vi "ma_SML RT Baseband Zoom FFT (real input).vi"(0 "x [V]":dbl[](array[numeric]) format="%.2f", 5 "zoom settings":T2={"zoom"=1, "stop band attenuation"=enum."120 dB", "alias protect in final transition"=FALSE, "oversampling ratio"=1.0} {"oversampling ratio" format="%.2f"; "zoom" min=0}, 7 "FFT settings":T3={"window"=1, "Window Size"=1024, "FFT Size"=1024, "%overlap"=0.0} {"%overlap" min=0.0 max=100.0 format="%.2f"; "window" items=["Rectangle"=0, "Hanning"=1, "Hamming"=2, "Blackman-Harris"=3, "Exact Blackman"=4, "Blackman"=5, "Flat Top"=6, "4 Term B-Harris "=7, "7 Term B-Harris"=8, "Low Sidelobe"=9, "Blackman Nuttall"=11, "Triangle"=30, "Bartlett-Hanning"=31, "Bohman"=32, "Parzen"=33, "Welch"=34, "Kaiser"=60, "Dolph-Chebyshev"=61, "Gaussian"=62]}, 11 "error in (no error)":errorcluster, 12 "reset?":bool) -> (4 "FFT{X} [Vrms]":cdb[](array[numeric]) format="%.2f", 6 "time data":dbl[](array[numeric]) format="%.2f", 8 "spectral info":T1 {"window" items=["Rectangle"=0, "Hanning"=1, "Hamming"=2, "Blackman-Harris"=3, "Exact Blackman"=4, "Blackman"=5, "Flat Top"=6, "4 Term B-Harris "=7, "7 Term B-Harris"=8, "Low Sidelobe"=9, "Blackman Nuttall"=11, "Triangle"=30, "Bartlett-Hanning"=31, "Bohman"=32, "Parzen"=33, "Welch"=34, "Kaiser"=60, "Dolph-Chebyshev"=61, "Gaussian"=62]}, 10 "spectrum ready?":bool, 14 "filter transition length":i32=1 min=0, 15 "error out":errorcluster)   [LabVIEW 2020, in "NI_MAPro.lvlib"]
uses:
  NI_MAPro.lvlib
  ma_sml_Spectral Info.ctl
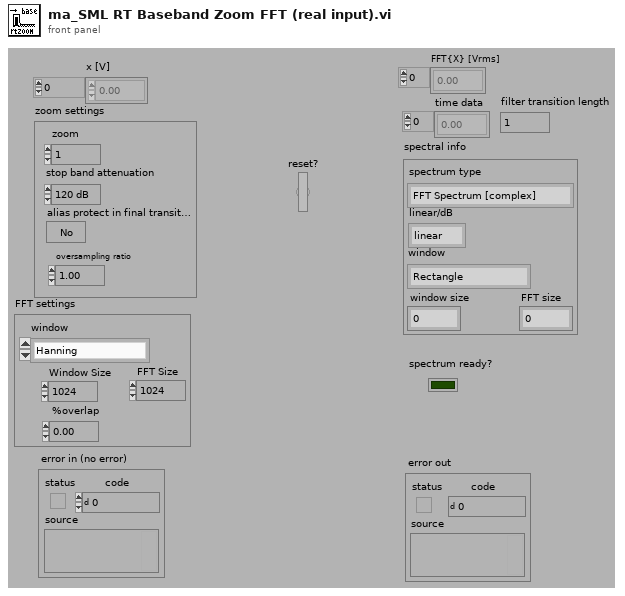
[diagram p1: front panel]
types:
  T1 = typedef "NI_MAPro.lvlib/ma_sml_Spectral Info.ctl" = cluster{"spectrum type":enum16{"FFT Spectrum [complex]", "Amplitude [Magnitude]", "Power [Magnitude^2]", "Cross Spectrum [complex]", "Frequency Response [Complex]"}, "linear/dB":enum16{"linear", "dB"}, "window":u16, "window size":i32, "FFT size":i32}
  T2 = cluster{"zoom":i32, "stop band attenuation":enum16{"84 dB", "96 dB", "120 dB"}, "alias protect in final transition":bool, "oversampling ratio":dbl}
  T3 = cluster{"window":u16, "Window Size":i32, "FFT Size":i32, "%overlap":dbl}
  T4 = cluster{"zoom":bool, "stop band attenuation":bool, "alias protect in final transition":bool, "oversampling ratio":bool}
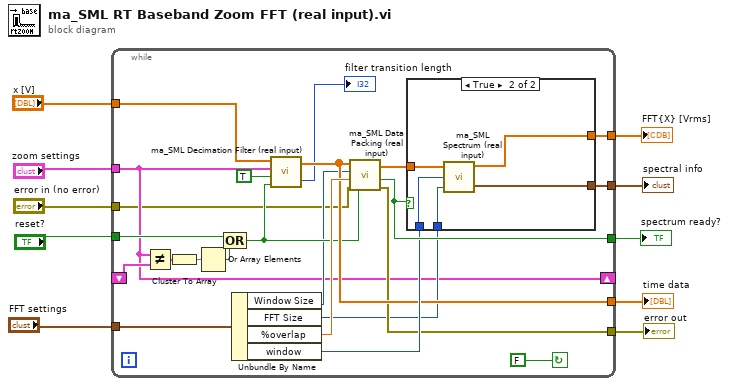
[diagram p0: block diagram]
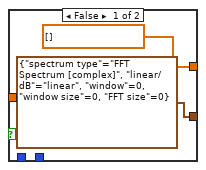
[diagram p2: hidden frame]
diagram:
  n1 = while {
    tunnel: [w11] -> w1
    tunnel: "reset?" -> [w26]
    tunnel: "error in (no error)" -> [w12]
    tunnel: "x [V]" -> [w13]
    tunnel: "FFT settings" -> [w14]
    tunnel: "zoom settings" -> [w15]
    tunnel: [w22] -> w7
    tunnel: [w23] -> w8
    tunnel: [w24] -> w9
    shift-left: _ -> [w25]
    shift-right: [w15] -> _
    tunnel: [w33] -> w10
    stop <- FALSE continue-if-true
    n2 = Not Equal?(x=w15, y=w25) -> (x != y?=w28:T4)
    n3 = Cluster To Array(cluster=w28) -> (array=w27:bool[])
    n4 = Or Array Elements(Boolean array=w27) -> (logical OR=w31:bool)
    n5 = Compound Arithmetic op=OR(w26, w31) -> (w21:bool)
    n6 = Unbundle By Name(w14) -> ("Window Size"=w18:i32, "FFT Size"=w17:i32, "%overlap"=w30:dbl, "window"=w29:u16)
    n7 = call "ma_SML Decimation Filter (real input).vi"("reset?"=w21, "truncate transition?"=TRUE ("Truncate initial filter Transition"), "decimation setting"=w15, "x"=w13) -> ("initial cutoff length"=→"filter transition length":i32, "y"=w24:dbl[])
    n8 = call "ma_SML Data Packing (real input).vi"("reset?"=w21, "error in (no error)"=w12, "%overlap"=w30, "size"=w18, "x"=w24) -> ("error out"=w23:errorcluster, "data ready?"=w33:bool, "y"=w32:dbl[])  [unwired: 4 in]
    n9 = case shown="True" w33 {
      tunnel: [cdb[] [] ("FFT{x} [Vrms]") w40] -> w22
      tunnel: w32 -> [_ w38]
      tunnel: w29 -> [_ w39]
      tunnel: w17 -> [_ w37]
      tunnel: [T1 {"spectrum type"=enum."FFT Spectrum [complex]", "linear/dB"=enum."linear", "window"=0, "window size"=0, "FFT size"=0} ("spectral info") w36] -> w11
      frame False {
      }
      frame True {
        n10 = call "ma_SML Spectrum (real input).vi"("FFT Size"=w37, "window"=w39, "x[V]"=w38) -> ("spectral info"=w36:T1, "FFT{x} [Vrms]"=w40:cdb[])
      }
    }
  }
  "spectrum ready?" <- w10
  "FFT{X} [Vrms]" <- w7
  "time data" <- w9
  "error out" <- w8
  "spectral info" <- w1
